vi "Query System LED.vi"(0 "VISA resource name":refnum<visa-resource-name>, 11 "error in (no error)":errorcluster) -> (4 "VISA resource name out":refnum<visa-resource-name>, 6 "LED Blinking":bool, 15 "error out":errorcluster)   [LabVIEW 2020, in "NH Research Regenerative Test Series.lvlib"]
doc: "Reports if the LED on the module is blinking or not."
uses:
  NH Research Regenerative Test Series.lvlib
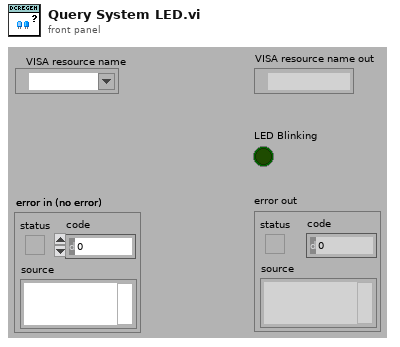
[diagram p1: front panel]
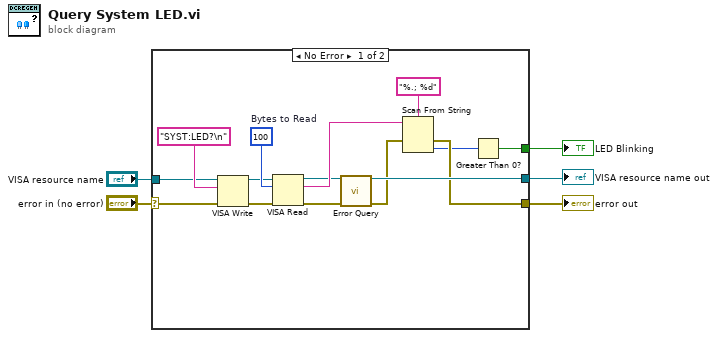
[diagram p0: block diagram]
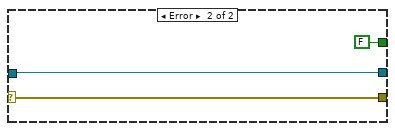
[diagram p2: hidden frame]
diagram:
  n1 = case shown="No Error" "error in (no error)" {
    selector: "error in (no error)" -> [w16 w23]
    tunnel: [w8 w23] -> w4
    tunnel: [w12 w22] -> w2
    tunnel: "VISA resource name" -> [w15 w22]
    tunnel: [w6 FALSE] -> w1
    frame No Error {
      w20 = u32 100  # Bytes to Read
      n2 = VISA Write(VISA resource name=w15, write buffer="SYST:LED?\n", error in (no error)=w16) -> (VISA resource name out=w18:refnum<visa-resource-name>, error out=w19:errorcluster)  [unwired: 1 out]
      n3 = VISA Read(VISA resource name=w18, byte count=w20, error in (no error)=w19) -> (VISA resource name out=w11:refnum<visa-resource-name>, read buffer=w14:string, error out=w10:errorcluster)  [unwired: 1 out]
      n4 = call "Error Query.vi"("VISA resource name"=w11, "error in (no error)"=w10) -> ("VISA resource name out"=w12:refnum<visa-resource-name>, "error out"=w9:errorcluster)  [unwired: 10 in, 2 out]
      n5 = Scan From String(format string="%.; %d", input string=w14, error in=w9) -> (error out=w8:errorcluster, output 1=w7:i32)  [unwired: 2 in, 2 out]
      n6 = Greater Than 0?(x=w7) -> (x > 0?=w6:bool)
    }
    frame Error {
    }
  }
  "error out" <- w4
  "VISA resource name out" <- w2
  "LED Blinking" <- w1
